vi "연속읽기요구(subVI).vi"(1 "직접변수(Byte)":string, 2 "데이터개수(Byte)":u16) -> (0 "연속읽기":string)   [LabVIEW 2014]
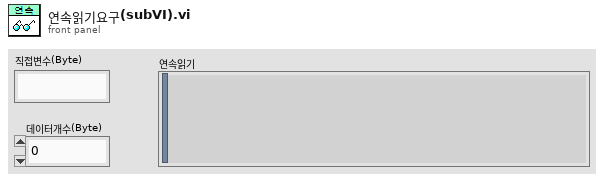
[diagram p1: front panel]
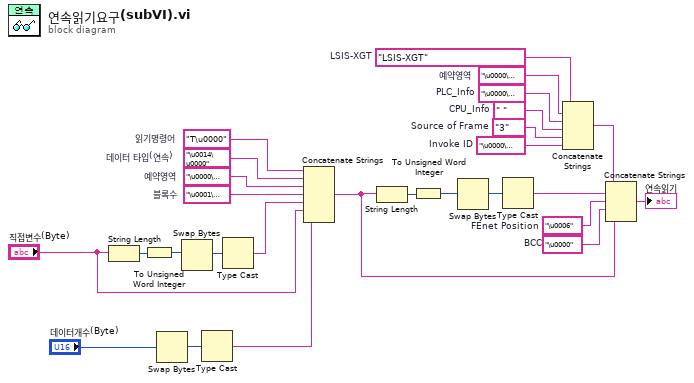
[diagram p0: block diagram]
diagram:
  w13 = "\u0001\u0000"  # 블록수
  w15 = "\u0000"  # BCC
  w1 = "\u0006"  # FEnet Position
  w18 = "\u0000\u0000"  # Invoke ID
  w19 = "3"  # Source of Frame
  w20 = " "  # CPU_Info
  w21 = "\u0000\u0000"  # PLC_Info
  w22 = "\u0000\u0000"  # 예약영역
  w23 = "LSIS-XGT"  # LSIS-XGT
  w25 = "\u0000\u0000"  # 예약영역
  w26 = "\u0014\u0000"  # 데이터 타입(연속)
  w27 = "T\u0000"  # 읽기명령어
  n1 = String Length(string="직접변수(Byte)") -> (length=w12:i32)
  n2 = To Unsigned Word Integer(number=w12) -> (unsigned 16bit integer=w6:u16)
  n3 = Swap Bytes(anything="데이터개수(Byte)") -> (byte swapped=w4:u16)
  n4 = Swap Bytes(anything=w6) -> (byte swapped=w7:u16)
  n5 = Type Cast(x=w4) -> (*(type *) &x=w3:string)  [unwired: 1 in]
  n6 = Type Cast(x=w7) -> (*(type *) &x=w5:string)  [unwired: 1 in]
  n7 = Concatenate Strings(w27, w26, w25, w13, w5, "직접변수(Byte)", w3) -> (w16:string)
  n8 = String Length(string=w16) -> (length=w24:i32)
  n9 = To Unsigned Word Integer(number=w24) -> (unsigned 16bit integer=w10:u16)
  n10 = Swap Bytes(anything=w10) -> (byte swapped=w9:u16)
  n11 = Type Cast(x=w9) -> (*(type *) &x=w8:string)  [unwired: 1 in]
  n12 = Concatenate Strings(w23, w22, w21, w20, w19, w18) -> (w17:string)
  n13 = Concatenate Strings(w17, w8, w1, w15, w16) -> (→"연속읽기":string)
